vi "WPILibLoadRecords.vi"(8 "error in (no error)":errorcluster, 10 "loading q":refnum<queue>, 11 "Data Value Reference in":refnum<data-value>) -> (0 "error out":errorcluster, 3 "Data Value Reference out":refnum<data-value>)   [LabVIEW 2020]
uses:
  Typedef/WPILibLog.ctl
  Typedef/Header.ctl
  Typedef/Entry.ctl
  Typedef/Record.ctl
  <vilib>/Utility/miscctls.llb/LVMapReplaceAction.ctl
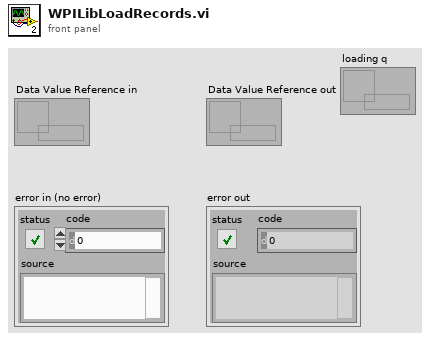
[diagram p1: front panel]
types:
  T1 = typedef "WPILibLog.ctl" = cluster{"Header":T2, "Record Start Idx":i32, "Entries":map{u32, T3}, "file ref":refnum<file>, "Finished Entries":T3[], "raw data":u8[]}
  T2 = typedef "Header.ctl" = cluster{"Header String":string, "Version":dbl, "Header Extra String Length":u32, "Header Extra String":string}
  T3 = typedef "Entry.ctl" = cluster{"ID":u32, "Records":T4[], "Finished?":bool, "Name":string, "Type":string, "Metadata":string, "RecordCnt":i32}
  T4 = typedef "Record.ctl" = cluster{"raw data":u8[], "ID":u32, "Size (bytes)":u32, "Timestamp":u64}
  T5 = enum16{"big-endian, network order", "native, host order", "little-endian"}
  T6 = typedef "LVMapReplaceAction.ctl" = enum32{"Modify Entry only if found", "Add or Modify Entry", "Delete Entry"}
  T7 = typedef "Control Header.ctl" = cluster{"Control Type":u8, "ID":u32, "Name Length":u32, "Name":string, "Type Length":u32, "Type":string, "Metadata Length":u32, "Metadata":string}
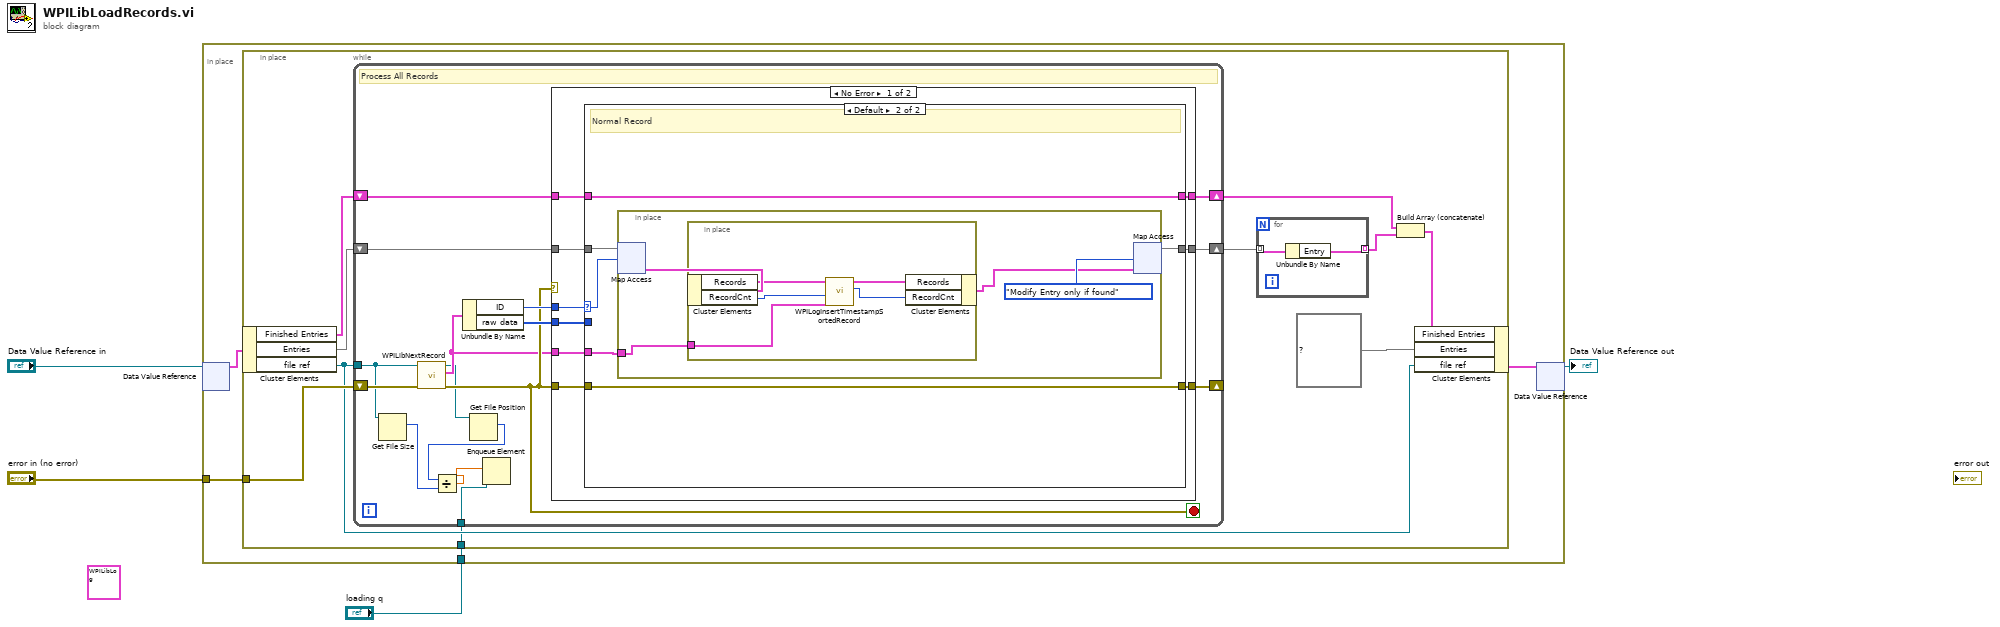
[diagram p0: block diagram]
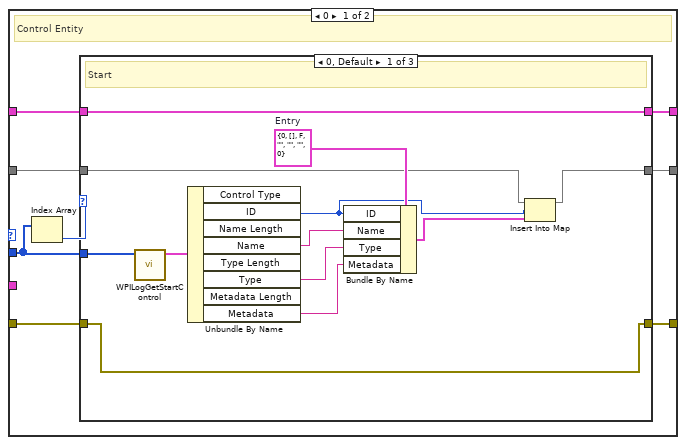
[diagram p2: hidden frame]
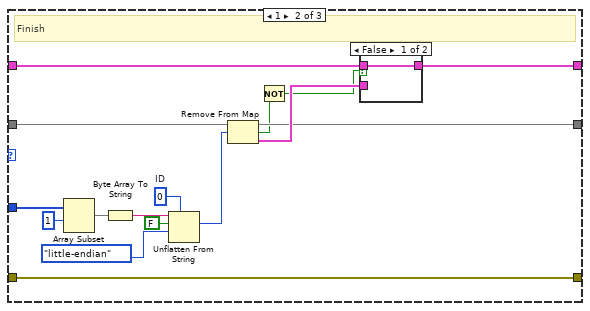
[diagram p3: hidden frame]
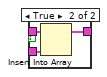
[diagram p4: hidden frame]
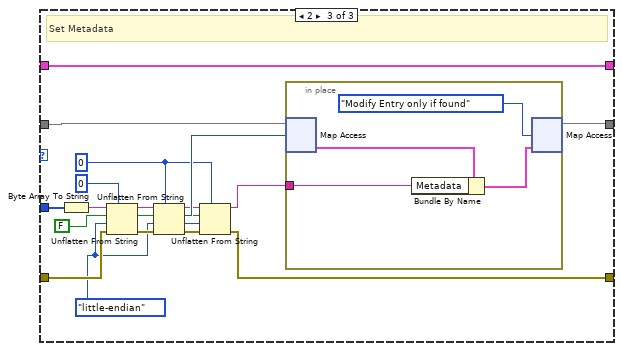
[diagram p5: hidden frame]
diagram:
  (unwired) T1 {"Header"={"Header String"="", "Version"=0.0, "Header Extra String Length"=0, "Header Extra String"=""}, "Record Start Idx"=0, "Entries"={}, "file ref"=refnum, "Finished Entries"=[], "raw data"=[]} ("data value")
  n1 = in-place {
    in-place-border: "error in (no error)" -> [w6]
    in-place-border: "loading q" -> [w5]
    n2 = in-place-dvr #1("Data Value Reference in") -> (w8:T1)  [unwired: 1 out]
    n3 = in-place {
      in-place-border: w6 -> [w18]
      in-place-border: w5 -> [w9]
      n4 = in-place-cluster #2(w8) -> ("Finished Entries"=w16:T3[], "Entries"=w17:map{u32, T3}, "file ref"=w15:refnum<file>)
      n5 = while {
        tunnel: w15 -> [w26]
        shift-right: [w35] -> _
        shift-left: w18 -> [w36]
        shift-right: [w31] -> w14
        shift-left: w17 -> [w33]
        shift-right: [w29] -> w12
        shift-left: w16 -> [w30]
        tunnel: w9 -> [w22]
        stop <- w28 stop-if-true
        # "Process All Records"
        n6 = Get File Size(file=w26) -> (size (in bytes)=w23:i64)  [unwired: 1 in, 2 out]
        n7 = call "WPILibNextRecord.vi"("error in (no error)"=w36, "Byte Stream File in"=w26) -> ("error out"=w28:errorcluster, "Record"=w27:T4, "refnum out"=w25:refnum<file>)  [unwired: 7 in]
        n8 = Unbundle By Name(w27) -> ("ID"=w34:u32, "raw data"=w32:u8[])
        n9 = Get File Position(7:w25) -> (2:w24:i64)  [unwired: 1 in, 2 out]
        n10 = Divide(x=w24, y=w23) -> (x/y=w21:dbl)
        n11 = Enqueue Element(queue=w22, element=w21) -> ()  [unwired: 2 in, 3 out]
        n12 = case shown="No Error" w28 {
          tunnel: [w45 w124] -> w35
          tunnel: w34 -> [w44 _]
          tunnel: w28 -> [w43 w124]
          tunnel: w33 -> [w42 w122]
          tunnel: w32 -> [w41 _]
          tunnel: [w40 w122] -> w31
          tunnel: w30 -> [w39 w123]
          tunnel: [w38 w123] -> w29
          tunnel: w27 -> [w37 _]
          frame No Error {
            n13 = case shown="Default" w44 {
              selector: w44 -> [_ w109]
              tunnel: w43 -> [w47 w112]
              tunnel: [w46 w112] -> w45
              tunnel: w42 -> [w53 w110]
              tunnel: w41 -> [w51 _]
              tunnel: [w50 w108] -> w40
              tunnel: w39 -> [w49 w111]
              tunnel: [w48 w111] -> w38
              tunnel: w37 -> [_ w107]
              frame 0 {
                # "Control Entity"
                n14 = Index Array(array=w51) -> (element=w52:u8)  [unwired: 1 in]
                n15 = case shown="0, Default" w52 {
                  tunnel: w53 -> [w59 w74 w101]
                  tunnel: w51 -> [w64 w78 w99]
                  tunnel: [w56 w70 w100] -> w50
                  tunnel: w49 -> [w55 w72 w102]
                  tunnel: [w55 w69 w102] -> w48
                  tunnel: w47 -> [w54 w66 w95]
                  tunnel: [w54 w66 w94] -> w46
                  frame 0, Default {
                    w63 = T3 {"ID"=0, "Records"=[], "Finished?"=FALSE, "Name"="", "Type"="", "Metadata"="", "RecordCnt"=0}  # Entry
                    # "Start"
                    n16 = call "WPILogGetStartControl.vi"("raw data"=w64) -> ("Control Entry"=w65:T7)  [unwired: 8 in, 2 out]
                    n17 = Unbundle By Name(w65) -> ("ID"=w58:u32, "Name"=w62:string, "Type"=w61:string, "Metadata"=w60:string)  [unwired: 4 out]
                    n18 = Bundle By Name(cluster=w63, "ID"=w58, "Name"=w62, "Type"=w61, "Metadata"=w60) -> (w57:T3)
                    n19 = Insert Into Map(map in=w59, key=w58, value=w57) -> (map out=w56:map{u32, T3})  [unwired: 2 out]
                  }
                  frame 1 {
                    w75 = u32 0  # ID
                    # "Finish"
                    n20 = Array Subset(array=w78, index=1) -> (w76:u8[])  [unwired: 1 in]
                    n21 = Byte Array To String(unsigned byte array=w76) -> (string=w81:string)
                    n22 = Unflatten From String(type=w75, binary string=w81, data includes array or string size? (T)=FALSE, byte order (0:big-endian, network order)=T5."little-endian") -> (value=w73:u32)  [unwired: 1 in, 2 out]
                    n23 = Remove From Map(10:w73, 11:w74) -> (1:w71:T3, 2:w68:bool, 3:w70:map{u32, T3})
                    n24 = Not(x=w68) -> (.not. x?=w67:bool)
                    n25 = case shown="False" w67 {
                      tunnel: w72 -> [w82 w85]
                      tunnel: w71 -> [_ w84]
                      tunnel: [w82 w83] -> w69
                      frame False {
                      }
                      frame True {
                        n26 = Insert Into Array(array=w85, new element=w84) -> (w83:T3[])  [unwired: 1 in]
                      }
                    }
                  }
                  frame 2 {
                    w87 = T5."little-endian" ("byte order (0:big-endian, network order)")
                    w88 = FALSE ("data includes array or string size? (T)")
                    w86 = u32 0
                    # "Set Metadata"
                    n27 = Byte Array To String(unsigned byte array=w99) -> (string=w98:string)
                    n28 = Unflatten From String(type=u8 0, binary string=w98, data includes array or string size? (T)=w88, byte order (0:big-endian, network order)=w87, error in (no error)=w95) -> (rest of the binary string=w89:string, error out=w97:errorcluster)  [unwired: 1 out]
                    n29 = Unflatten From String(type=w86, binary string=w89, data includes array or string size? (T)=w88, byte order (0:big-endian, network order)=w87, error in (no error)=w97) -> (rest of the binary string=w90:string, value=w92:u32, error out=w96:errorcluster)
                    n30 = Unflatten From String(type=w86, binary string=w90, data includes array or string size? (T)=w88, byte order (0:big-endian, network order)=w87, error in (no error)=w96) -> (rest of the binary string=w91:string, error out=w94:errorcluster)  [unwired: 1 out]
                    n31 = in-place {
                      in-place-border: w91 -> [w104]
                      n32 = in-place-map #3(w101, w92) -> (w105:T3)  [unwired: 1 in, 1 out]
                      n33 = Bundle By Name(cluster=w105, "Metadata"=w104) -> (w103:T3)
                      n34 = in-place-map #3(w103, LVMapReplaceAction."Modify Entry only if found" ("action")) -> (w100:map{u32, T3})  [unwired: 2 out]
                    }
                  }
                }
              }
              frame Default {
                # "Normal Record"
                n35 = in-place {
                  in-place-border: w107 -> [w113]
                  n36 = in-place-map #4(w110, w109) -> (w115:T3)  [unwired: 1 in, 1 out]
                  n37 = in-place {
                    in-place-border: w113 -> [w119]
                    n38 = in-place-cluster #5(w115) -> ("Records"=w121:T4[], "RecordCnt"=w117:i32)
                    n39 = call "WPILogInsertTimestampSortedRecord.vi"("SizeIn"=w117, "Record"=w119, "Records"=w121) -> ("SizeOut"=w118:i32, "Array"=w120:T4[])  [unwired: 7 in]
                    n40 = in-place-cluster #5("Records"=w120, "RecordCnt"=w118) -> (w114:T3)
                  }
                  n41 = in-place-map #4(w114, LVMapReplaceAction."Modify Entry only if found" ("action")) -> (w108:map{u32, T3})  [unwired: 2 out]
                }
              }
            }
          }
          frame Error {
          }
        }
      }
      n42 = for {
        tunnel: [w19] -> w13 mode=indexing
        tunnel: w14 -> [w20] mode=indexing
        n43 = Unbundle By Name(w20) -> ("Entry"=w19:T3)
      }
      n44 = Build Array (concatenate)(w12, w13) -> (w11:T3[])
      n45 = in-place-cluster #2("Finished Entries"=w11, "Entries"=map{u32, T3} {}, "file ref"=w15) -> (w7:T1)
    }
    n46 = in-place-dvr #1(w7) -> (→"Data Value Reference out":refnum<data-value>)  [unwired: 1 out]
  }
